vi "Update Chart Legend State.vi"(10 "Enabled?":bool, 11 "WaveformChart in":refnum<vi>) -> (0 "error out":errorcluster)   [LabVIEW 2014, in "Chart Module.lvlib"]
uses:
  Chart Module.lvlib
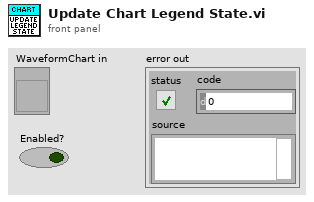
[diagram p1: front panel]
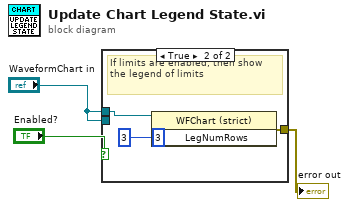
[diagram p0: block diagram]
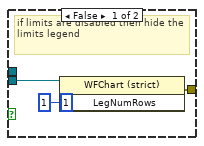
[diagram p2: hidden frame]
diagram:
  n1 = case shown="True" "Enabled?" {
    tunnel: [w6 w9] -> w3
    tunnel: "WaveformChart in" -> [w5 _]
    tunnel: "WaveformChart in" -> [_ w8]
    frame False {
      (unwired) u32 1 ("Legend:Number of Rows")
      # "if limits are disabled then hide the limits legend"
      n2 = property on="Property Node" class="WFChart (strict)"(reference=w5, "LegNumRows"=u32 1 ("Legend:Number of Rows")) -> (error out=w6:errorcluster)  [unwired: 1 in, 1 out]
    }
    frame True {
      (unwired) u32 3 ("Legend:Number of Rows")
      # "If limits are enabled, then show  the legend of limits"
      n3 = property on="Property Node" class="WFChart (strict)"(reference=w8, "LegNumRows"=u32 3 ("Legend:Number of Rows")) -> (error out=w9:errorcluster)  [unwired: 1 in, 1 out]
    }
  }
  "error out" <- w3
